vi "Configure Trigger.vi"(6 "Trigger Slope (0: Positive)":u16(ring) items=["Positive", "Negative", "Either"], 7 "Trigger Source (0: Immediate)":u16(ring) items=["Immediate", "Internal", "External", "Software Trigger Function"], 8 "error in (no error)":errorcluster, 9 "Trigger Mode (0: Edge)":u16(ring) items=["Edge", "Level"], 10 "Channel (1: Channel1)":u16(ring)=1 items=["Channel1"=1, "Channel2"=2], 11 "VISA resource name":refnum<visa-resource-name>) -> (0 "error out":errorcluster, 3 "VISA resource name out":refnum<visa-resource-name>)   [LabVIEW 2009, in "Agilent 81150.lvlib"]
doc: "Configures the trigger source for triggering sweeps.\n\n<B>Note(s):</B>\nUse this VI only with other low-level VIs. The high-level VIs automatically incorporate this functionality. This VI does not check the instrument status. If you want to check the instrument status, call the Error Query VI at the conclusion of your sweep operation."
uses:
  Agilent 81150.lvlib
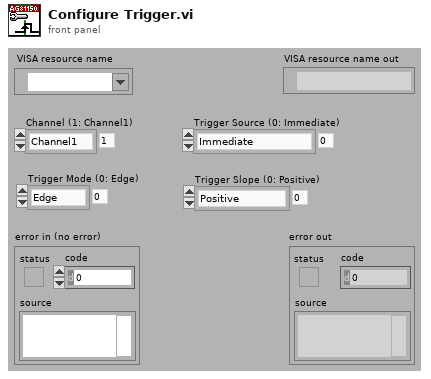
[diagram p1: front panel]
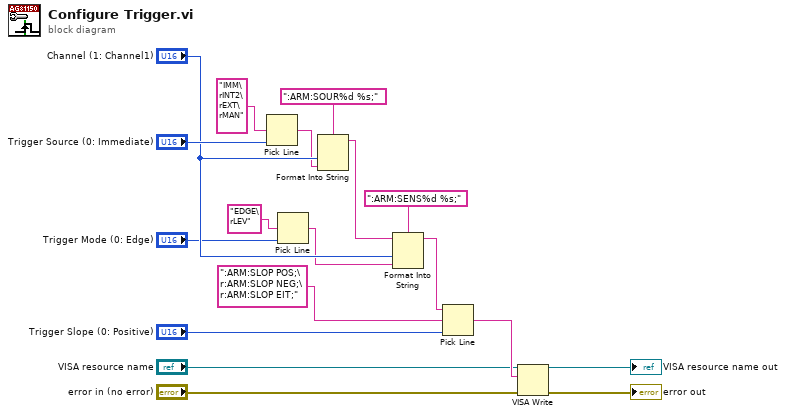
[diagram p0: block diagram]
diagram:
  n1 = Pick Line(multi-line string="IMM\rINT2\rEXT\rMAN", line index="Trigger Source (0: Immediate)") -> (output string=w14:string)  [unwired: 1 out]
  n2 = Pick Line(multi-line string="EDGE\rLEV", line index="Trigger Mode (0: Edge)") -> (output string=w9:string)  [unwired: 1 out]
  n3 = Format Into String(format string=":ARM:SOUR%d %s;", "Channel (1: Channel1)", w14) -> (resulting string=w10:string)  [unwired: 2 in, 1 out]
  n4 = Format Into String(format string=":ARM:SENS%d %s;", initial string=w10, "Channel (1: Channel1)", w9) -> (resulting string=w8:string)  [unwired: 1 in, 1 out]
  n5 = Pick Line(string ("")=w8, multi-line string=":ARM:SLOP POS;\r:ARM:SLOP NEG;\r:ARM:SLOP EIT;", line index="Trigger Slope (0: Positive)") -> (output string=w5:string)
  n6 = VISA Write(VISA resource name="VISA resource name", write buffer=w5, error in (no error)="error in (no error)") -> (VISA resource name out=→"VISA resource name out":refnum<visa-resource-name>, error out=→"error out":errorcluster)  [unwired: 1 out]
